vi "globalTearDown.vi"(8 "error in (no error)":errorcluster, 11 "testcase-CSMSubModule in":refnum<class "testcase-CSMSubModule.lvclass">) -> (0 "error out":errorcluster, 3 "testcase-CSMSubModule out":refnum<class "testcase-CSMSubModule.lvclass">)   [LabVIEW 2017, in "testcase-CSMSubModule.lvclass"]
uses:
  testcase-CSMSubModule.lvclass
  testcase-CSMSubModule.lvclass/testcase-CSMSubModule.ctl
  <vilib>/addons/_JKI Toolkits/VI Tester/TestCase.llb/TestCase.lvclass
  src/user.lib/_NEVSTOP/Communicable State Machine(CSM)/_Support/Typedef/_CSM_List Module Scope.ctl
  src/user.lib/_NEVSTOP/Communicable State Machine(CSM)/Communicable State Machine.lvlib
panel:
  out "Module Names":string[](array[string])
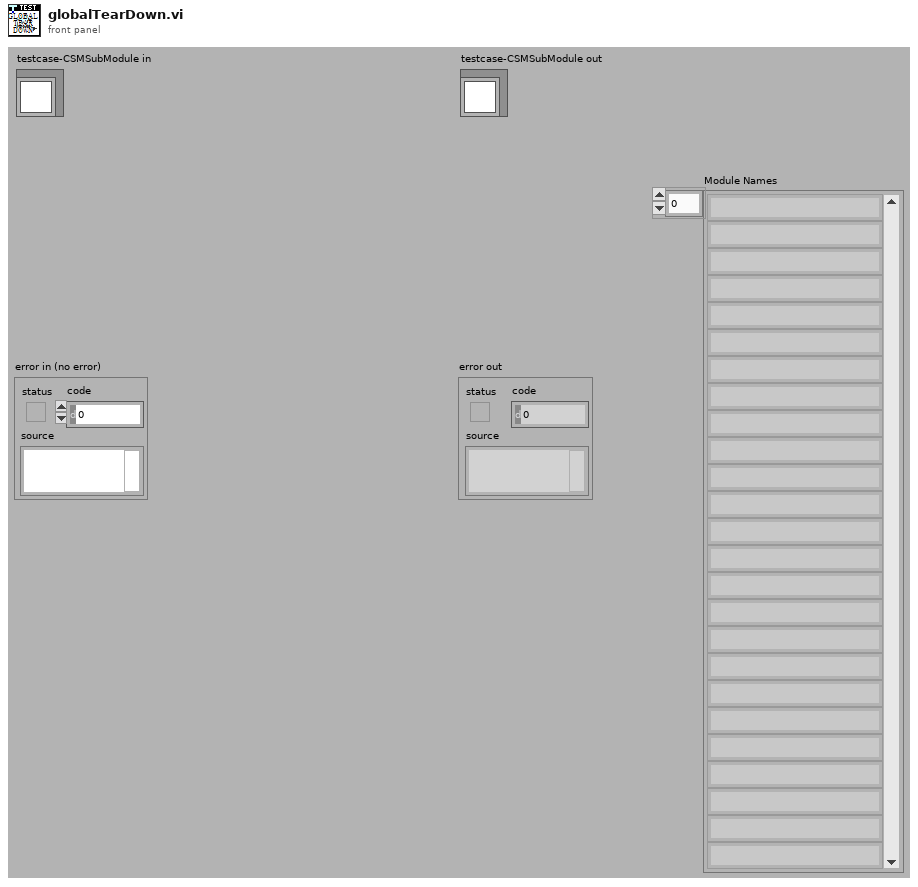
[diagram p1: front panel]
types:
  T1 = typedef "Communicable State Machine.lvlib/_CSM_List Module Scope.ctl" = enum16{"Normal", "System Only", "All"}
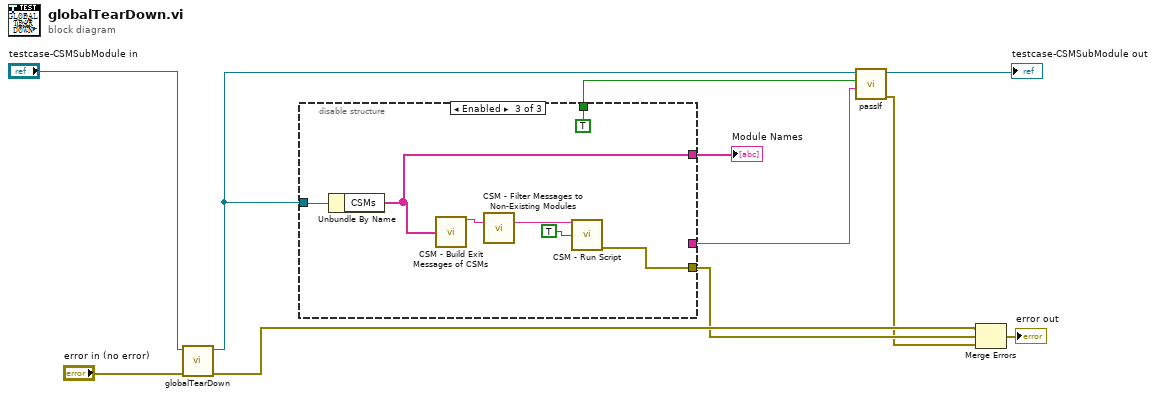
[diagram p0: block diagram]
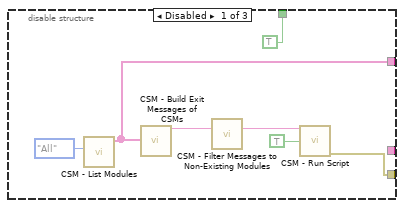
[diagram p2: hidden frame]
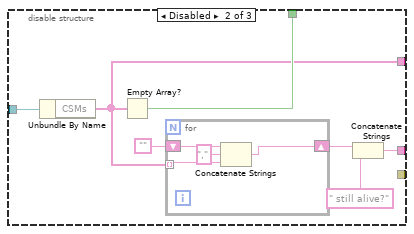
[diagram p3: hidden frame]
diagram:
  n1 = call-parent "globalTearDown.vi"("error in (no error)"="error in (no error)", "TestCase in"="testcase-CSMSubModule in") -> ("error out"=w5:errorcluster, "TestCase out"=w1:refnum<class "testcase-CSMSubModule.lvclass">)  [unwired: 8 in]
  n2 = disable-structure shown="Enabled" {
    disable-tunnel: [w14 _ w31] -> w4
    disable-tunnel: w1 -> [_ w25 w36]
    disable-tunnel: [w13 w23 w32] -> w8
    disable-tunnel: [TRUE w24 TRUE ("pass")] -> w7
    disable-tunnel: [_ w19 _] -> w6
    frame Disabled {
      n3 = call "CSM - List Modules.vi"("Scope (Normal)"=_CSM_List_Module_Scope."All") -> ("Module Names"=w13:string[])  [unwired: 9 in, 1 out]
      n4 = call "CSM - Build Exit Messages of CSMs.vi"("CSMs"=w13) -> ("States"=w18:string)  [unwired: 14 in]
      n5 = call "CSM - Filter Messages to Non-Existing Modules.vi"("States In"=w18) -> ("States Out"=w16:string)  [unwired: 14 in]
      n6 = call "CSM - Run Script.vi"("CSM Scripts"=w16, "Continue If Error? (F)"=TRUE) -> ("error out"=w14:errorcluster)  [unwired: 11 in, 2 out]
    }
    frame Disabled {
      n7 = Unbundle By Name(w25) -> ("CSMs"=w23:string[])
      n8 = Empty Array?(array=w23) -> (empty?=w24:bool)
      n9 = for {
        tunnel: w23 -> [w27] mode=indexing
        shift-right: [w28] -> w21
        shift-left: "" -> [w29]
        n10 = Concatenate Strings(w29, "," ("string"), w27) -> (w28:string)
      }
      n11 = Concatenate Strings(w21, " still alive?" ("string")) -> (w19:string)
    }
    frame Enabled {
      n12 = Unbundle By Name(w36) -> ("CSMs"=w32:string[])
      n13 = call "CSM - Build Exit Messages of CSMs.vi"("CSMs"=w32) -> ("States"=w35:string)  [unwired: 14 in]
      n14 = call "CSM - Filter Messages to Non-Existing Modules.vi"("States In"=w35) -> ("States Out"=w33:string)  [unwired: 14 in]
      n15 = call "CSM - Run Script.vi"("CSM Scripts"=w33, "Continue If Error? (F)"=TRUE) -> ("error out"=w31:errorcluster)  [unwired: 11 in, 2 out]
    }
  }
  "Module Names" <- w8
  n16 = call-dynamic "passIf.vi"("message (\"\")"=w6, "pass"=w7, "TestCase in"=w1) -> ("error out"=w3:errorcluster, "TestCase out"=→"testcase-CSMSubModule out":refnum<class "testcase-CSMSubModule.lvclass">)  [unwired: 7 in]
  n17 = Merge Errors(w5, w4, w3) -> (→"error out":errorcluster)
